vi "FXP NIPLL_OnePoleARM_IIR.vi"(1 "alpha [U16.0]":fxp<+,16,0>, 3 "x":fxp<+/-,32,3>) -> (0 "y[n]":fxp<+/-,48,3>)   [LabVIEW 2009]
uses:
  <vilib>/rvi/FXPMathLib/FxpMul/XNode/nifxpmath_Multiplier.xnode
  <vilib>/rvi/FXPMathLib/FxpMul/subVIs/nifxpmath_Mul_SimConfig.ctl
  <vilib>/fxp/LVFixedPointQuantizationPolicyTypeDef.ctl
  <vilib>/fxp/LVFixedPointOverflowPolicyTypeDef.ctl
  <vilib>/rvi/FXPMathLib/FxpMul/simVIs/DllFxpMulTemp_sub.vi
  <vilib>/rvi/FXPMathLib/FxpAdd/XNode/nifxpmath_Add.xnode
  <vilib>/rvi/FXPMathLib/FxpAdd/subVIs/nifxpmath_Add_SimConfig.ctl
  <vilib>/rvi/FXPMathLib/FxpAdd/simVIs/DllFxpAddTemp_sub.vi
panel:
  # "Pole location: 1-alpha\nH[z] = alpha/(1-z^-1 * (1-alpha))"
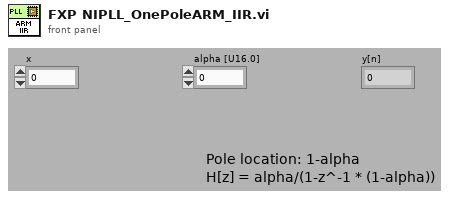
[diagram p1: front panel]
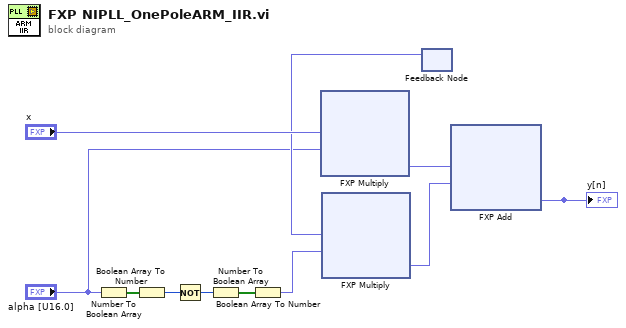
[diagram p0: block diagram]
diagram:
  n1 = Number To Boolean Array(number="alpha [U16.0]") -> (Boolean array=w6:bool[])
  n2 = Boolean Array To Number(Boolean array=w6) -> (number=w5:u16)
  n3 = Not(x=w5) -> (.not. x?=w4:u16)
  n4 = Number To Boolean Array(number=w4) -> (Boolean array=w3:bool[])
  n5 = Boolean Array To Number(Boolean array=w3) -> (number=w1:fxp<+,16,0>)
  n6 = xnode "FXP Multiply"("x"="x", "y"="alpha [U16.0]") -> ("x*y"=w10:fxp<+/-,48,3>)
  n7 = feedback #1() -> (w7:fxp<+/-,48,3>)  [unwired: 1 in]
  n8 = xnode "FXP Multiply"("x"=w7, "y"=w1) -> ("x*y"=w9:fxp<+/-,48,3>)
  n9 = xnode "FXP Add"("x"=w10, "y"=w9) -> ("x+y"=w8:fxp<+/-,48,3>)
  "y[n]" <- w8
